vi "FL_LvInterface.vi"() -> ()   [LabVIEW 2011]
panel:
  in  "LibUSB Device VID/PID":string="1443:0007"
  in  "Tab Control":T1(tab)
  in  "xsvf file":path=path "T:/FpgaLinkDemo.xsvf"
  in  "Play":bool
  in  "Channel to Read":u8
  in  "Bytes to Read":u32=1
  in  "Timeout (10000)":u32=10000
  out "Data Read":u8[](array[numeric]) format="%.0x"
  in  "Read":bool
  in  "Write":bool
  in  "Data to Write":u8[](array[numeric]) format="%.0x"
  in  "Write Timeout (10000)":u32=10000
  in  "Channel to Write":u8
  in  "Channel to Read":u8
  in  "Timeout ms (2 mins)":u32=120000
  in  "Read File":bool
  in  "Write File":bool
  in  "Timeout ms (2 mins)":u32=120000
  in  "Channel to Write":u8
  in  "Write to FPGA from file":path=path "T:/testWrite.bin"
  in  "Read from FPGA to file":path=path "T:/testRead.bin"
  in  "Bytes to Read":u32=1
  out "File Result":string
  in  "Scan":bool
  out "Device List":u32[](array[numeric]) format="%.0x"
  out "Number of Devices Found":u32
  in  "stop":bool
  out "Exit error out":errorcluster
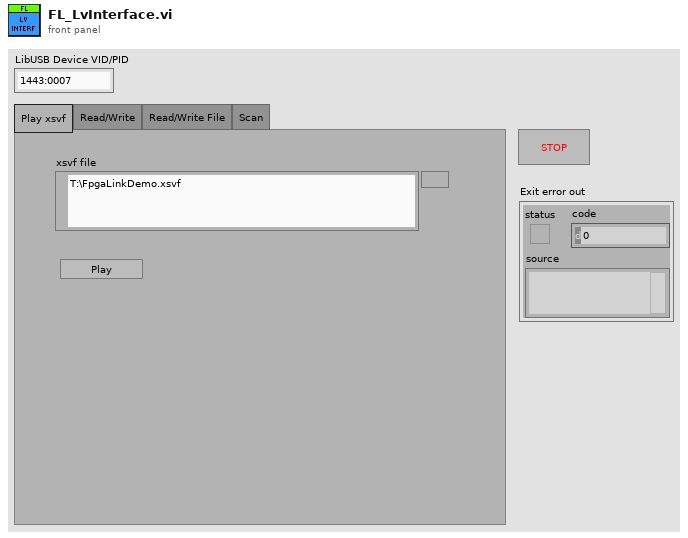
[diagram p1: front panel]
types:
  T1 = enum32{"Play xsvf", "Read/Write", "Read/Write File", "Scan"}
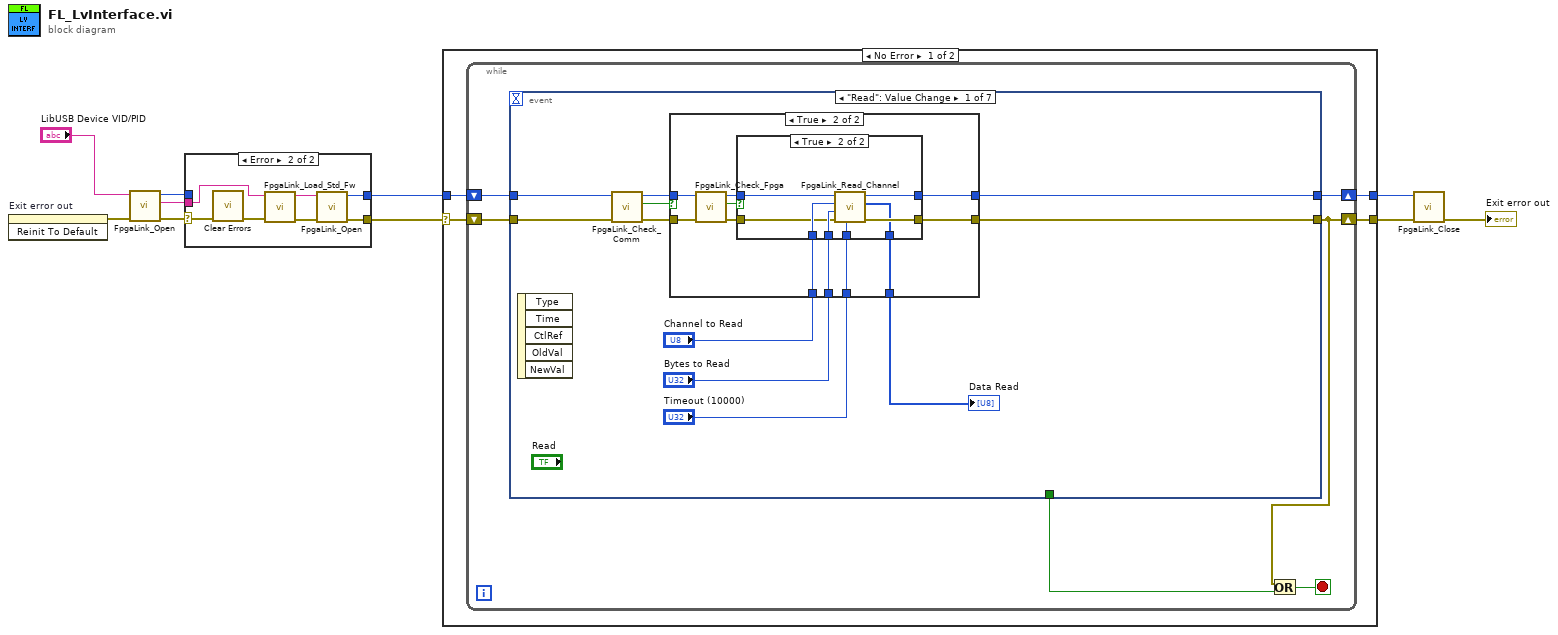
[diagram p0: block diagram]
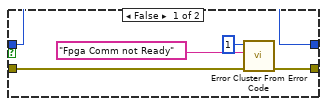
[diagram p2: hidden frame]
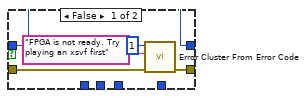
[diagram p3: hidden frame]
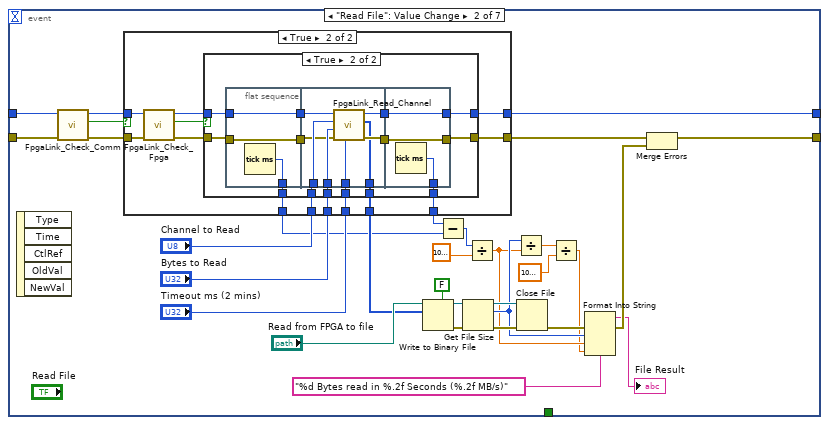
[diagram p4: hidden frame]
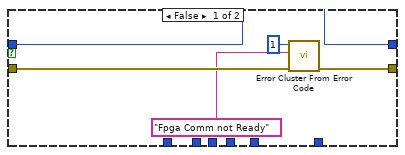
[diagram p5: hidden frame]
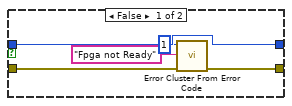
[diagram p6: hidden frame]
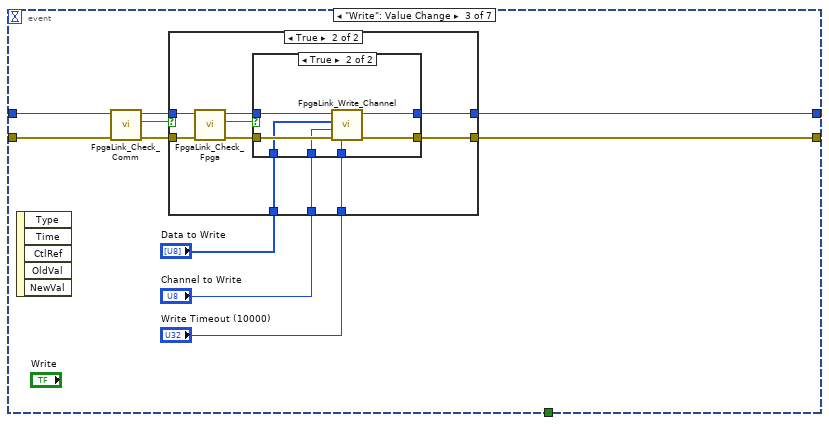
[diagram p7: hidden frame]
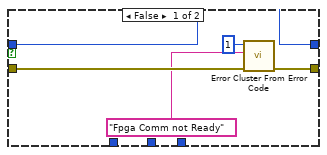
[diagram p8: hidden frame]
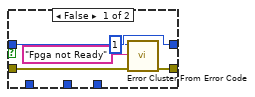
[diagram p9: hidden frame]
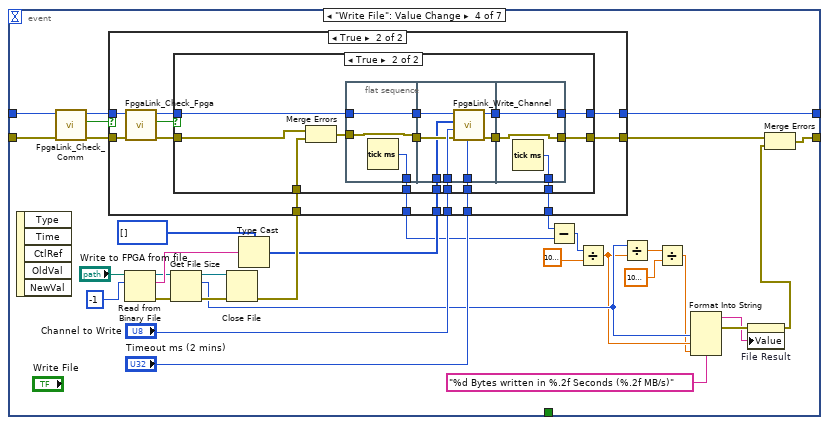
[diagram p10: hidden frame]
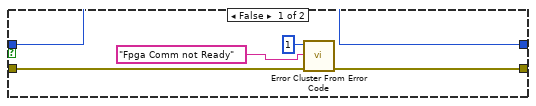
[diagram p11: hidden frame]
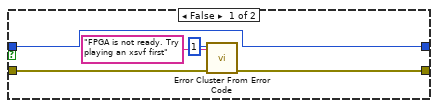
[diagram p12: hidden frame]
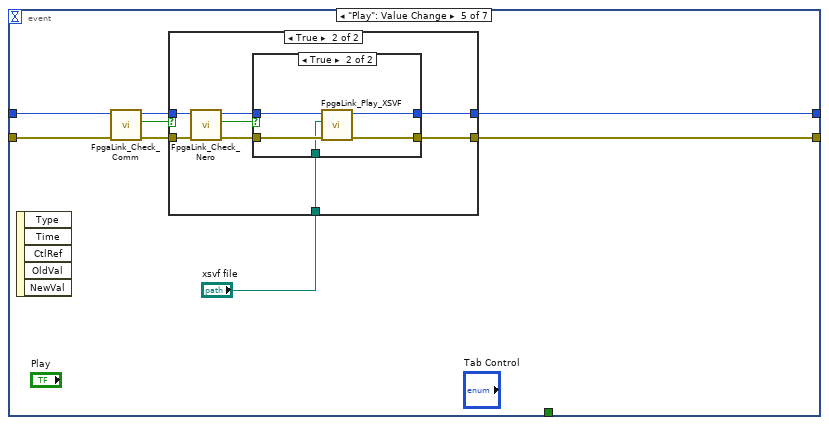
[diagram p13: hidden frame]
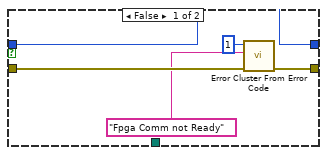
[diagram p14: hidden frame]
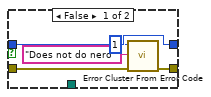
[diagram p15: hidden frame]
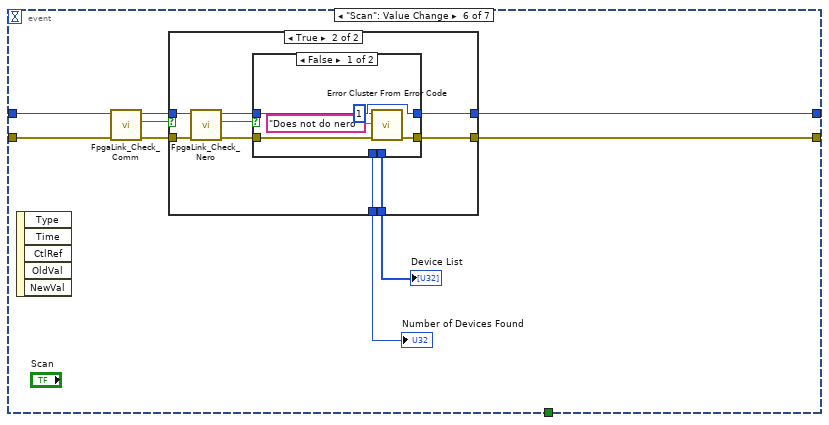
[diagram p16: hidden frame]
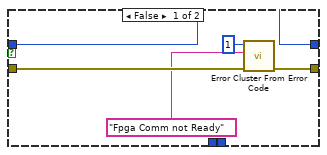
[diagram p17: hidden frame]
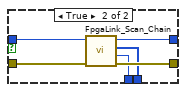
[diagram p18: hidden frame]
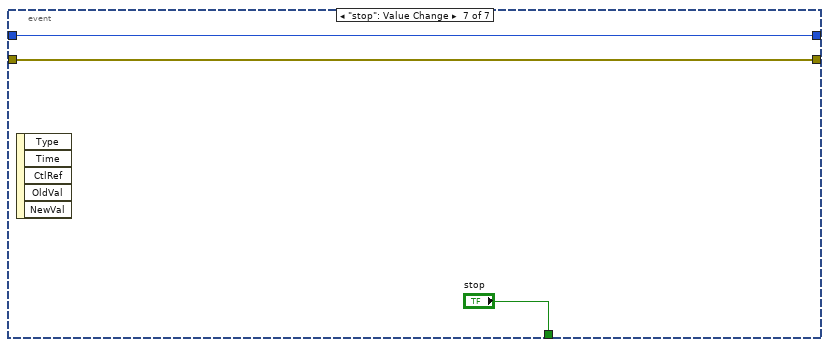
[diagram p19: hidden frame]
diagram:
  n1 = invoke on="Exit error out" class="Clust (strict)" method="Reinit To Default"() -> (error out=w1:errorcluster)  [unwired: 3 in, 2 out]
  n2 = call <vilib>:"FpgaLink_Open.vi"("error in (no error)"=w1, "VP"="LibUSB Device VID/PID") -> ("error out"=w9:errorcluster, "VP Out"=w6:string, "handle out"=w7:i64)  [unwired: 7 in]
  n3 = case shown="Error" w9 {
    selector: w9 -> [w12 w14]
    tunnel: [w12 w18] -> w2
    tunnel: w7 -> [w11 _]
    tunnel: [w11 w16] -> w5
    tunnel: w6 -> [_ w15]
    frame No Error {
    }
    frame Error {
      n4 = call <vilib>:"Clear Errors.vi"("error in (no error)"=w14) -> ("error out"=w13:errorcluster)  [unwired: 6 in]
      n5 = call <vilib>:"FpgaLink_Load_Std_Fw.vi"("error in (no error)"=w13, "VP"=w15) -> ("error out"=w19:errorcluster, "New VP"=w17:string)  [unwired: 8 in]
      n6 = call <vilib>:"FpgaLink_Open.vi"("error in (no error)"=w19, "VP"=w17) -> ("error out"=w18:errorcluster, "handle out"=w16:i64)  [unwired: 7 in, 1 out]
    }
  }
  n7 = case shown="No Error" w2 {
    selector: w2 -> [w20 w342]
    tunnel: w5 -> [w23 w341]
    tunnel: [w22 w341] -> w4
    tunnel: [w21 w342] -> w3
    frame No Error {
      n8 = while {
        shift-right: [w27] -> w22
        shift-left: w23 -> [w29]
        shift-right: [w25] -> w21
        shift-left: w20 -> [w28]
        stop <- w26 stop-if-true
        n9 = event shown="[0] \"Read\": Value Change" {
          selector: _ -> [_ _ _ _ _ _ _]
          dyn-events: _ -> [_ _ _ _ _ _ _]
          timeout: _ -> [_ _ _ _ _ _ _]
          tunnel: w29 -> [w32 w97 w155 w218 w276 w308 w339]
          tunnel: w28 -> [w34 w99 w157 w220 w278 w310 w340]
          tunnel: [w37 w100 w159 w221 w280 w312 w339] -> w27
          tunnel: [w36 w90 w158 w191 w279 w311 w340] -> w25
          tunnel: [_ _ _ _ _ _ "stop"] -> w24
          event "Read": Value Change {
            n10 = event-data() -> ()  [unwired: 1 in, 5 out]
            n11 = call <vilib>:"FpgaLink_Check_Comm.vi"("error in (no error)"=w34, "handle"=w32) -> ("error out"=w33:errorcluster, "Is Capable?"=w30:bool, "handle out"=w31:i64)  [unwired: 7 in]
            n12 = case shown="True" w30 {
              tunnel: "Channel to Read" -> [_ w56]
              tunnel: "Bytes to Read" -> [_ w55]
              tunnel: "Timeout (10000)" -> [_ w54]
              tunnel: [w45 w53] -> w37
              tunnel: [w43 w52] -> w36
              tunnel: [_ w51] -> w35
              tunnel: w33 -> [w44 w50]
              tunnel: w31 -> [w45 w49]
              frame False {
                n13 = call <vilib>:"Error Cluster From Error Code.vi"("error in (no error)"=w44, "error message (\"\")"="Fpga Comm not Ready" ("error message (\"\")"), "error code (0)"=1) -> ("error out"=w43:errorcluster)  [unwired: 6 in]
              }
              frame True {
                n14 = call <vilib>:"FpgaLink_Check_Fpga.vi"("error in (no error)"=w50, "handle"=w49) -> ("error out"=w48:errorcluster, "Is Running?"=w47:bool, "handle out"=w46:i64)  [unwired: 7 in]
                n15 = case shown="True" w47 {
                  tunnel: w56 -> [_ w69]
                  tunnel: w55 -> [_ w68]
                  tunnel: w54 -> [_ w67]
                  tunnel: [w61 w66] -> w53
                  tunnel: [w59 w65] -> w52
                  tunnel: [_ w64] -> w51
                  tunnel: w48 -> [w60 w63]
                  tunnel: w46 -> [w61 w62]
                  frame False {
                    n16 = call <vilib>:"Error Cluster From Error Code.vi"("error in (no error)"=w60, "error message (\"\")"="FPGA is not ready. Try playing an xsvf first" ("error message (\"\")"), "error code (0)"=1) -> ("error out"=w59:errorcluster)  [unwired: 6 in]
                  }
                  frame True {
                    n17 = call <vilib>:"FpgaLink_Read_Channel.vi"("Timeout (10000)"=w67, "error in (no error)"=w63, "Count"=w68, "Channel"=w69, "handle"=w62) -> ("error out"=w65:errorcluster, "data"=w64:u8[], "handle out"=w66:i64)  [unwired: 4 in]
                  }
                }
              }
            }
            "Data Read" <- w35
          }
          event "Read File": Value Change {
            n18 = event-data() -> ()  [unwired: 1 in, 5 out]
            n19 = call <vilib>:"FpgaLink_Check_Comm.vi"("error in (no error)"=w99, "handle"=w97) -> ("error out"=w98:errorcluster, "Is Capable?"=w95:bool, "handle out"=w96:i64)  [unwired: 7 in]
            n20 = case shown="True" w95 {
              tunnel: "Channel to Read" -> [_ w118]
              tunnel: "Bytes to Read" -> [_ w117]
              tunnel: "Timeout ms (2 mins)" -> [_ w116]
              tunnel: [w105 w115] -> w100
              tunnel: [w103 w114] -> w91
              tunnel: [_ w113] -> w92
              tunnel: w98 -> [w104 w112]
              tunnel: w96 -> [w105 w111]
              tunnel: [_ w107] -> w85
              tunnel: [_ w106] -> w86
              frame False {
                n21 = call <vilib>:"Error Cluster From Error Code.vi"("error in (no error)"=w104, "error message (\"\")"="Fpga Comm not Ready" ("error message (\"\")"), "error code (0)"=1) -> ("error out"=w103:errorcluster)  [unwired: 6 in]
              }
              frame True {
                n22 = call <vilib>:"FpgaLink_Check_Fpga.vi"("error in (no error)"=w112, "handle"=w111) -> ("error out"=w110:errorcluster, "Is Running?"=w109:bool, "handle out"=w108:i64)  [unwired: 7 in]
                n23 = case shown="True" w109 {
                  tunnel: w118 -> [_ w137]
                  tunnel: w117 -> [_ w136]
                  tunnel: w116 -> [_ w135]
                  tunnel: [w123 w134] -> w115
                  tunnel: [w121 w133] -> w114
                  tunnel: [_ w126] -> w113
                  tunnel: w110 -> [w122 w132]
                  tunnel: w108 -> [w123 w131]
                  tunnel: [_ w125] -> w107
                  tunnel: [_ w124] -> w106
                  frame False {
                    n24 = call <vilib>:"Error Cluster From Error Code.vi"("error in (no error)"=w122, "error message (\"\")"="Fpga not Ready" ("error message (\"\")"), "error code (0)"=1) -> ("error out"=w121:errorcluster)  [unwired: 6 in]
                  }
                  frame True {
                    n25 = flat-sequence {
                      tunnel: w131 -> [w139]
                      tunnel: w132 -> [w140]
                      tunnel: [w140] -> w130
                      tunnel: [w139] -> w129
                      tunnel: [w138] -> w125
                      tunnel: w137 -> [w148]
                      tunnel: w136 -> [w147]
                      tunnel: w135 -> [w146]
                      tunnel: w130 -> [w143]
                      tunnel: w129 -> [w142]
                      tunnel: [w145] -> w128
                      tunnel: [w144] -> w127
                      tunnel: [w141] -> w126
                      tunnel: [w150] -> w133
                      tunnel: [w151] -> w134
                      tunnel: w128 -> [w151]
                      tunnel: w127 -> [w150]
                      tunnel: [w149] -> w124
                      frame #0 {
                        n26 = Tick Count (ms)() -> (millisecond timer value=w138:u32)
                      }
                      frame #1 {
                        n27 = call <vilib>:"FpgaLink_Read_Channel.vi"("Timeout (10000)"=w146, "error in (no error)"=w143, "Count"=w147, "Channel"=w148, "handle"=w142) -> ("error out"=w144:errorcluster, "data"=w141:u8[], "handle out"=w145:i64)  [unwired: 4 in]
                      }
                      frame #2 {
                        n28 = Tick Count (ms)() -> (millisecond timer value=w149:u32)
                      }
                    }
                  }
                }
              }
            }
            n29 = Write to Binary File(file (use dialog)="Read from FPGA to file", data=w92, 5:FALSE ("prepend array or string size? (T)")) -> (refnum out=w84:refnum<file>, error out=w83:errorcluster)  [unwired: 3 in, 1 out]
            n30 = Subtract(x=w86, y=w85) -> (x-y=w76:u32)
            n31 = Get File Size(file=w84, error in=w83) -> (refnum out=w81:refnum<file>, size (in bytes)=w74:i64, 0:w82:errorcluster)
            n32 = Divide(x=w76, y=1000.0) -> (x/y=w73:dbl)
            n33 = Divide(x=w74, y=w73) -> (x/y=w72:dbl)
            n34 = Close File(refnum=w81, error in=w82) -> (error out=w80:errorcluster)  [unwired: 1 out]
            n35 = Divide(x=w72, y=1000000.0) -> (x/y=w70:dbl)
            n36 = Format Into String(format string="%d Bytes read in %.2f Seconds (%.2f MB/s)", error in=w80, w74, w73, w70) -> (resulting string=→"File Result":string, error out=w79:errorcluster)  [unwired: 1 in]
            n37 = Merge Errors(w91, w79) -> (w90:errorcluster)
          }
          event "Write": Value Change {
            n38 = event-data() -> ()  [unwired: 1 in, 5 out]
            n39 = call <vilib>:"FpgaLink_Check_Comm.vi"("error in (no error)"=w157, "handle"=w155) -> ("error out"=w156:errorcluster, "Is Capable?"=w153:bool, "handle out"=w154:i64)  [unwired: 7 in]
            n40 = case shown="True" w153 {
              tunnel: "Channel to Write" -> [_ w176]
              tunnel: "Write Timeout (10000)" -> [_ w175]
              tunnel: [w166 w174] -> w159
              tunnel: [w164 w173] -> w158
              tunnel: w156 -> [w165 w172]
              tunnel: w154 -> [w166 w171]
              tunnel: "Data to Write" -> [_ w167]
              frame False {
                n41 = call <vilib>:"Error Cluster From Error Code.vi"("error in (no error)"=w165, "error message (\"\")"="Fpga Comm not Ready" ("error message (\"\")"), "error code (0)"=1) -> ("error out"=w164:errorcluster)  [unwired: 6 in]
              }
              frame True {
                n42 = call <vilib>:"FpgaLink_Check_Fpga.vi"("error in (no error)"=w172, "handle"=w171) -> ("error out"=w170:errorcluster, "Is Running?"=w169:bool, "handle out"=w168:i64)  [unwired: 7 in]
                n43 = case shown="True" w169 {
                  tunnel: w176 -> [_ w183]
                  tunnel: w175 -> [_ w182]
                  tunnel: [w181 w185] -> w174
                  tunnel: [w179 w188] -> w173
                  tunnel: w170 -> [w180 w187]
                  tunnel: w168 -> [w181 w186]
                  tunnel: w167 -> [_ w184]
                  frame False {
                    n44 = call <vilib>:"Error Cluster From Error Code.vi"("error in (no error)"=w180, "error message (\"\")"="Fpga not Ready" ("error message (\"\")"), "error code (0)"=1) -> ("error out"=w179:errorcluster)  [unwired: 6 in]
                  }
                  frame True {
                    n45 = call <vilib>:"FpgaLink_Write_Channel.vi"("Timeout (10000)"=w182, "error in (no error)"=w187, "Channel"=w183, "data"=w184, "handle"=w186) -> ("error out"=w188:errorcluster, "handle out"=w185:i64)  [unwired: 5 in]
                  }
                }
              }
            }
          }
          event "Write File": Value Change {
            n46 = event-data() -> ()  [unwired: 1 in, 5 out]
            n47 = call <vilib>:"FpgaLink_Check_Comm.vi"("error in (no error)"=w220, "handle"=w218) -> ("error out"=w219:errorcluster, "Is Capable?"=w216:bool, "handle out"=w217:i64)  [unwired: 7 in]
            n48 = Read from Binary File(10:-1 ("count (1)"), 11:"Write to FPGA from file") -> (0:w209:errorcluster, 2:w211:string, 3:w206:refnum<file>)  [unwired: 4 in, 1 out]
            n49 = Get File Size(file=w206, error in=w209) -> (refnum out=w207:refnum<file>, size (in bytes)=w197:i64, 0:w208:errorcluster)
            n50 = Close File(refnum=w207, error in=w208) -> (error out=w212:errorcluster)  [unwired: 1 out]
            n51 = Type Cast(type=u8[] [] ("data"), x=w211) -> (*(type *) &x=w201:u8[])
            n52 = case shown="True" w216 {
              tunnel: "Channel to Write" -> [_ w239]
              tunnel: "Timeout ms (2 mins)" -> [_ w238]
              tunnel: [w226 w237] -> w221
              tunnel: [w224 w236] -> w192
              tunnel: w219 -> [w225 w235]
              tunnel: w217 -> [w226 w234]
              tunnel: w212 -> [_ w230]
              tunnel: w201 -> [_ w229]
              tunnel: [_ w228] -> w200
              tunnel: [_ w227] -> w199
              frame False {
                n53 = call <vilib>:"Error Cluster From Error Code.vi"("error in (no error)"=w225, "error message (\"\")"="Fpga Comm not Ready" ("error message (\"\")"), "error code (0)"=1) -> ("error out"=w224:errorcluster)  [unwired: 6 in]
              }
              frame True {
                n54 = call <vilib>:"FpgaLink_Check_Fpga.vi"("error in (no error)"=w235, "handle"=w234) -> ("error out"=w233:errorcluster, "Is Running?"=w232:bool, "handle out"=w231:i64)  [unwired: 7 in]
                n55 = case shown="True" w232 {
                  tunnel: w239 -> [_ w256]
                  tunnel: w238 -> [_ w252]
                  tunnel: [w244 w257] -> w237
                  tunnel: [w242 w259] -> w236
                  tunnel: w233 -> [w243 w255]
                  tunnel: w231 -> [w244 w258]
                  tunnel: w230 -> [_ w253]
                  tunnel: w229 -> [_ w249]
                  tunnel: [_ w248] -> w228
                  tunnel: [_ w245] -> w227
                  frame False {
                    n56 = call <vilib>:"Error Cluster From Error Code.vi"("error in (no error)"=w243, "error message (\"\")"="FPGA is not ready. Try playing an xsvf first" ("error message (\"\")"), "error code (0)"=1) -> ("error out"=w242:errorcluster)  [unwired: 6 in]
                  }
                  frame True {
                    n57 = Merge Errors(w255, w253) -> (w254:errorcluster)
                    n58 = flat-sequence {
                      tunnel: w254 -> [w261]
                      tunnel: w258 -> [w262]
                      tunnel: [w262] -> w251
                      tunnel: [w261] -> w250
                      tunnel: [w260] -> w248
                      tunnel: w256 -> [w266]
                      tunnel: w252 -> [w264]
                      tunnel: w251 -> [w268]
                      tunnel: w250 -> [w265]
                      tunnel: w249 -> [w263]
                      tunnel: [w269] -> w247
                      tunnel: [w267] -> w246
                      tunnel: [w271] -> w257
                      tunnel: [w272] -> w259
                      tunnel: w247 -> [w272]
                      tunnel: w246 -> [w271]
                      tunnel: [w270] -> w245
                      frame #0 {
                        n59 = Tick Count (ms)() -> (millisecond timer value=w260:u32)
                      }
                      frame #1 {
                        n60 = call <vilib>:"FpgaLink_Write_Channel.vi"("Timeout (10000)"=w264, "error in (no error)"=w265, "Channel"=w266, "data"=w263, "handle"=w268) -> ("error out"=w269:errorcluster, "handle out"=w267:i64)  [unwired: 5 in]
                      }
                      frame #2 {
                        n61 = Tick Count (ms)() -> (millisecond timer value=w270:u32)
                      }
                    }
                  }
                }
              }
            }
            n62 = Subtract(x=w199, y=w200) -> (x-y=w205:u32)
            n63 = Divide(x=w205, y=1000.0) -> (x/y=w196:dbl)
            n64 = Divide(x=w197, y=w196) -> (x/y=w203:dbl)
            n65 = Divide(x=w203, y=1000000.0) -> (x/y=w195:dbl)
            n66 = Format Into String(format string="%d Bytes written in %.2f Seconds (%.2f MB/s)", w197, w196, w195) -> (resulting string=w193:string, error out=w194:errorcluster)  [unwired: 2 in]
            n67 = property on="File Result" class="Str"(error in=w194, "Value"=w193) -> (error out=w190:errorcluster)  [unwired: 1 in, 1 out]
            n68 = Merge Errors(w192, w190) -> (w191:errorcluster)
          }
          event "Play": Value Change {
            n69 = event-data() -> ()  [unwired: 1 in, 5 out]
            n70 = call <vilib>:"FpgaLink_Check_Comm.vi"("error in (no error)"=w278, "handle"=w276) -> ("error out"=w277:errorcluster, "Is Capable?"=w274:bool, "handle out"=w275:i64)  [unwired: 7 in]
            n71 = case shown="True" w274 {
              tunnel: [w285 w293] -> w280
              tunnel: [w283 w292] -> w279
              tunnel: w277 -> [w284 w291]
              tunnel: w275 -> [w285 w289]
              tunnel: "xsvf file" -> [_ w286]
              frame False {
                n72 = call <vilib>:"Error Cluster From Error Code.vi"("error in (no error)"=w284, "error message (\"\")"="Fpga Comm not Ready" ("error message (\"\")"), "error code (0)"=1) -> ("error out"=w283:errorcluster)  [unwired: 6 in]
              }
              frame True {
                n73 = call <vilib>:"FpgaLink_Check_Nero.vi"("error in (no error)"=w291, "handle"=w289) -> ("error out"=w290:errorcluster, "Is Compatible?"=w287:bool, "handle out"=w288:i64)  [unwired: 7 in]
                n74 = case shown="True" w287 {
                  tunnel: [w298 w301] -> w293
                  tunnel: [w296 w302] -> w292
                  tunnel: w290 -> [w297 w303]
                  tunnel: w288 -> [w298 w300]
                  tunnel: w286 -> [_ w299]
                  frame False {
                    n75 = call <vilib>:"Error Cluster From Error Code.vi"("error in (no error)"=w297, "error message (\"\")"="Does not do nero" ("error message (\"\")"), "error code (0)"=1) -> ("error out"=w296:errorcluster)  [unwired: 6 in]
                  }
                  frame True {
                    n76 = call <vilib>:"FpgaLink_Play_XSVF.vi"("error in (no error)"=w303, "xsvf file"=w299, "handle"=w300) -> ("error out"=w302:errorcluster, "handle out"=w301:i64)  [unwired: 7 in]
                  }
                }
              }
            }
          }
          event "Scan": Value Change {
            n77 = event-data() -> ()  [unwired: 1 in, 5 out]
            n78 = call <vilib>:"FpgaLink_Check_Comm.vi"("error in (no error)"=w310, "handle"=w308) -> ("error out"=w309:errorcluster, "Is Capable?"=w306:bool, "handle out"=w307:i64)  [unwired: 7 in]
            n79 = case shown="True" w306 {
              tunnel: [w317 w326] -> w312
              tunnel: [w315 w325] -> w311
              tunnel: w309 -> [w316 w324]
              tunnel: w307 -> [w317 w322]
              tunnel: [_ w319] -> w305
              tunnel: [_ w318] -> w304
              frame False {
                n80 = call <vilib>:"Error Cluster From Error Code.vi"("error in (no error)"=w316, "error message (\"\")"="Fpga Comm not Ready" ("error message (\"\")"), "error code (0)"=1) -> ("error out"=w315:errorcluster)  [unwired: 6 in]
              }
              frame True {
                n81 = call <vilib>:"FpgaLink_Check_Nero.vi"("error in (no error)"=w324, "handle"=w322) -> ("error out"=w323:errorcluster, "Is Compatible?"=w320:bool, "handle out"=w321:i64)  [unwired: 7 in]
                n82 = case shown="False" w320 {
                  tunnel: [w331 w334] -> w326
                  tunnel: [w329 w337] -> w325
                  tunnel: w323 -> [w330 w336]
                  tunnel: w321 -> [w331 w335]
                  tunnel: [_ w333] -> w319
                  tunnel: [_ w332] -> w318
                  frame False {
                    n83 = call <vilib>:"Error Cluster From Error Code.vi"("error in (no error)"=w330, "error message (\"\")"="Does not do nero" ("error message (\"\")"), "error code (0)"=1) -> ("error out"=w329:errorcluster)  [unwired: 6 in]
                  }
                  frame True {
                    n84 = call <vilib>:"FpgaLink_Scan_Chain.vi"("error in (no error)"=w336, "handle"=w335) -> ("error out"=w337:errorcluster, "Number of Devices"=w332:u32, "Devices"=w333:u32[], "handle out"=w334:i64)  [unwired: 6 in]
                  }
                }
              }
            }
            "Device List" <- w305
            "Number of Devices Found" <- w304
          }
          event "stop": Value Change {
            n85 = event-data() -> ()  [unwired: 1 in, 5 out]
          }
        }
        n86 = Or(x=w25, y=w24) -> (x .or. y?=w26:bool)
      }
    }
    frame Error {
      # "Attempt to close handle anyway"
    }
  }
  n87 = call <vilib>:"FpgaLink_Close.vi"("error in (no error)"=w3, "handle"=w4) -> ("error out"=→"Exit error out":errorcluster)  [unwired: 9 in]
